vi "Do.vi"(8 "error in (no error)":errorcluster, 10 "Actor in":refnum<class "Actor.lvclass">, 11 "Send Software Advanced Trigger [AT] Msg":refnum<class "Send Software Advanced Trigger [AT] Msg.lvclass">) -> (0 "error out":errorcluster, 2 "Actor out":refnum<class "Actor.lvclass">)   [LabVIEW 2015, in "CS++Fgen.lvlib" / "Send Software Advanced Trigger [AT] Msg.lvclass"]
doc: "This VI delivers the message to the actor by calling the appropriate method(s) on the actor."
uses:
  Send Software Advanced Trigger [AT] Msg.lvclass
  <vilib>/ActorFramework/Actor/Actor.lvclass
  CS++Fgen/CS++Fgen.lvclass
  CSPP_Core/Actors/CS++PVMonitor Messages/CS++PVUpdate Msg/CS++PVUpdate Msg.lvclass/CS++PVUpdate Msg.ctl
  CSPP_Core/Classes/CS++ProcessVariables/ProcessVariable/PV.lvclass/PV.ctl
  Send Software Advanced Trigger [AT] Msg.lvclass/Send Software Advanced Trigger [AT] Msg.ctl
  CSPP_Core/Classes/CS++ProcessVariables/ProcessVariable/PV.lvclass
  CSPP_Core/Actors/CS++PVMonitor Messages/CS++PVUpdate Msg/CS++PVUpdate Msg.lvclass
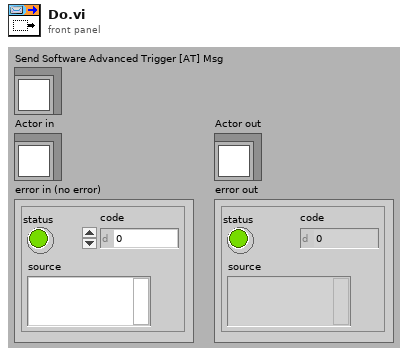
[diagram p1: front panel]
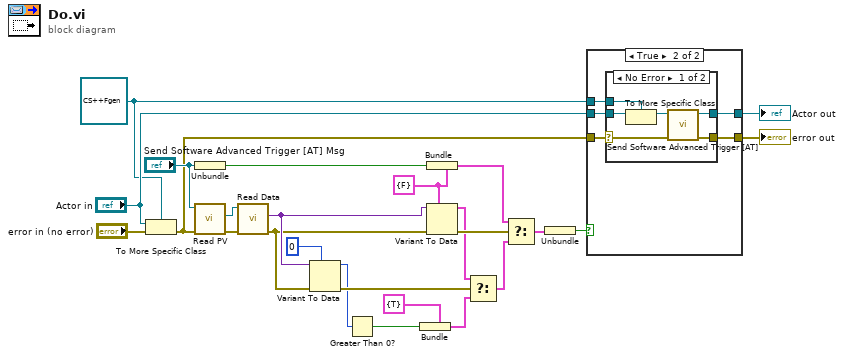
[diagram p0: block diagram]
diagram:
  w17 = cluster{bool} {FALSE} ("Type")
  w21 = refnum<class "CS++Fgen.lvclass"> refnum ("Actor in")
  n1 = To More Specific Class(target class=w21, reference="Actor in", error in="error in (no error)") -> (error out=w7:errorcluster)  [unwired: 1 out]
  n2 = Unbundle ("Pre-Unbundler")("Send Software Advanced Trigger [AT] Msg") -> (w1:bool)
  n3 = call "Read PV.vi"("error in (no error)"=w7, "CS++PVUpdate Msg in"="Send Software Advanced Trigger [AT] Msg") -> ("error out"=w20:errorcluster, "PV"=w16:refnum<class "PV.lvclass">)  [unwired: 7 in, 1 out]
  n4 = call "Read Data.vi"("error in (no error)"=w20, "PV in"=w16) -> ("error out"=w13:errorcluster, "Data"=w14:variant)  [unwired: 7 in, 1 out]
  n5 = Variant To Data ("I16-Conversion")(error in=w13, type=i16 0 ("I16-Conversion-Constant"), Variant=w14) -> (data=w6:i16, error out=w11:errorcluster)
  n6 = Greater Than 0? ("I16-Comp0")(x=w6) -> (x > 0?=w4:bool)
  n7 = Bundle ("I16-Bundle")(cluster=cluster{bool} {TRUE} ("I16-Cluster"), w4) -> (w3:cluster{bool})
  n8 = Bundle ("Pre-Bundler")(cluster=w17, w1) -> (w18:cluster{bool})
  n9 = Variant To Data(error in=w13, type=w17, Variant=w14) -> (data=w10:cluster{bool}, error out=w19:errorcluster)
  n10 = Select ("I16-Select")(t=w10, s=w11, f=w3) -> (s? t:f=w9:cluster{bool})
  n11 = Select ("MainSelect")(t=w18, s=w19, f=w9) -> (s? t:f=w12:cluster{bool})
  n12 = Unbundle ("Main-Unbundler")(w12) -> (w2:bool)
  n13 = case "Execute?" shown="True" w2 {
    tunnel: [w26 w32] -> w24
    tunnel: [w27 w31] -> w23
    tunnel: "Actor in" -> [w27 w30]
    tunnel: w21 -> [_ w29]
    tunnel: w7 -> [w26 w28]
    frame False {
    }
    frame True {
      n14 = case shown="No Error" w28 {
        selector: w28 -> [w36 w40]
        tunnel: [w38 w40] -> w32
        tunnel: [w37 w39] -> w31
        tunnel: w30 -> [w35 w39]
        tunnel: w29 -> [w34 _]
        frame No Error {
          n15 = To More Specific Class(target class=w34, reference=w35) -> (specific class reference=w33:refnum<class "CS++Fgen.lvclass">)  [unwired: 1 in, 1 out]
          n16 = call "Send Software Advanced Trigger [AT].vi"("error in (no error)"=w36, "CS++Fgen in"=w33) -> ("error out"=w38:errorcluster, "CS++Fgen out"=w37:refnum<class "CS++Fgen.lvclass">)  [unwired: 8 in]
        }
        frame Error {
        }
      }
    }
  }
  "error out" <- w24
  "Actor out" <- w23
